vi "Test.Pub.vi"() -> ()   [LabVIEW 2014]
panel:
  in  "stop":bool
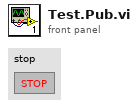
[diagram p1: front panel]
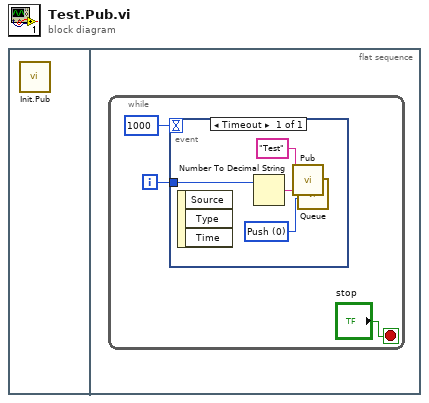
[diagram p0: block diagram]
diagram:
  n1 = flat-sequence {
    frame #0 {
      n2 = call "Init.Pub.vi"() -> ()  [unwired: 2 in, 1 out]
    }
    frame #1 {
      n3 = while {
        i -> [w1]
        stop <- "stop" stop-if-true
        n4 = event shown="[0] Timeout" {
          selector: _ -> [_]
          dyn-events: _ -> [_]
          timeout: 1000 -> [_]
          tunnel: w1 -> [w7]
          event Timeout {
            w4 = u16 0 items=["Push", "Pop"] ("Mode")
            w6 = "Test" ("Topic")
            n5 = event-data() -> ()  [unwired: 1 in, 3 out]
            n6 = Number To Decimal String(number=w7) -> (decimal integer string=w5:string)  [unwired: 1 in]
            n7 = call "Pub.vi"("Data"=w5, "Topic"=w6) -> ()  [unwired: 1 in, 1 out]
            n8 = call "Queue.vi"("Mode"=w4, "Value In"=w5, "Name"=w6) -> ()  [unwired: 1 in, 1 out]
          }
        }
      }
    }
  }
